vi "Global 1.vi"() -> ()   [LabVIEW 2018]
panel:
  in  "Numeric 4":dbl
  in  "Numeric 3":dbl
  in  "Numeric 2":dbl
  in  "Numeric":dbl
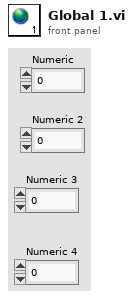
[diagram p1: front panel]
diagram:
